vi "Config Key String to DBL Array.vi"(7 "Section In":string, 8 "Error In":errorcluster, 10 "Key In":string, 11 "Ref In":T1) -> (0 "Error Out":errorcluster, 2 "1D DBL Array Out":dbl[](array[numeric]) format="%#_f", 3 "Ref Out":T1)   [LabVIEW 2024]
uses:
  <vilib>/Utility/config.llb/Config Data RefNum.ctl
  <vilib>/Utility/config.llb/Read Key (String).vi
  Converter/String To 1D DBL.vi
  <vilib>/Utility/config.llb/NI_LVConfig.lvlib
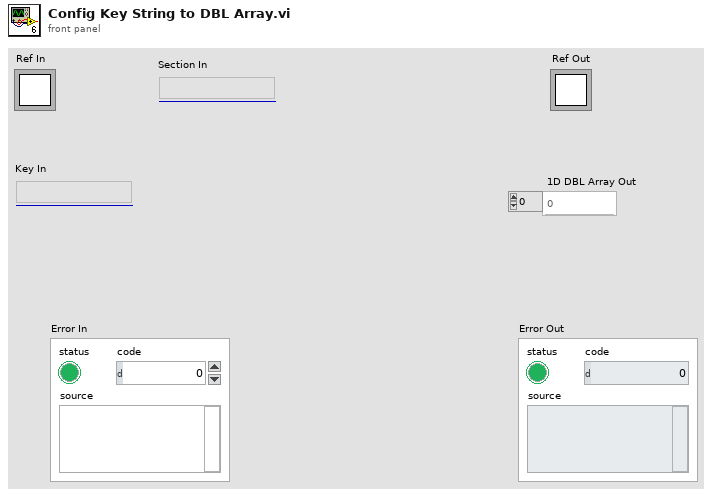
[diagram p1: front panel]
types:
  T1 = typedef "NI_LVConfig.lvlib/Config Data RefNum.ctl" = refnum<k1>
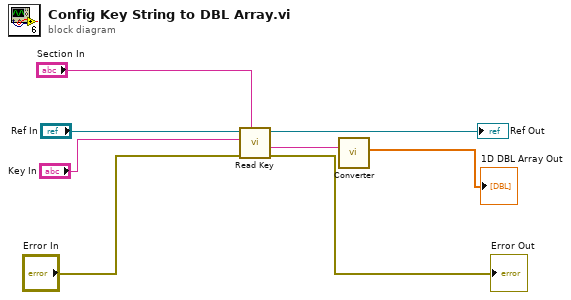
[diagram p0: block diagram]
diagram:
  n1 = call-poly <vilib>:"Read Key.vi"("section"="Section In", "error in (no error)"="Error In", "key"="Key In", "refnum"="Ref In") -> ("error out"=→"Error Out":errorcluster, "value"=w4:string, "refnum out"=→"Ref Out":T1)  [unwired: 4 in, 1 out]
  n2 = call-poly "Converter.vi"("String In"=w4) -> ("1D DBL Out"=→"1D DBL Array Out":dbl[])  [unwired: 10 in]
